vi "convertFromString.vi"(0 "reference in":refnum<class "Notification Controller.lvclass">, 5 "dateString":string, 7 "ICU?":bool, 9 "getDate":bool, 11 "error in (no error)":errorcluster, 12 "yearly?":bool, 13 "k4b2?":bool) -> (4 "reference out":refnum<class "Notification Controller.lvclass">, 6 "date":timestamp, 10 "send?":bool, 15 "error out":errorcluster)   [LabVIEW 2014, in "Notification Controller.lvclass"]
uses:
  Notification Controller.lvclass
  <vilib>/Utility/miscctls.llb/LVDateTimeRec.ctl
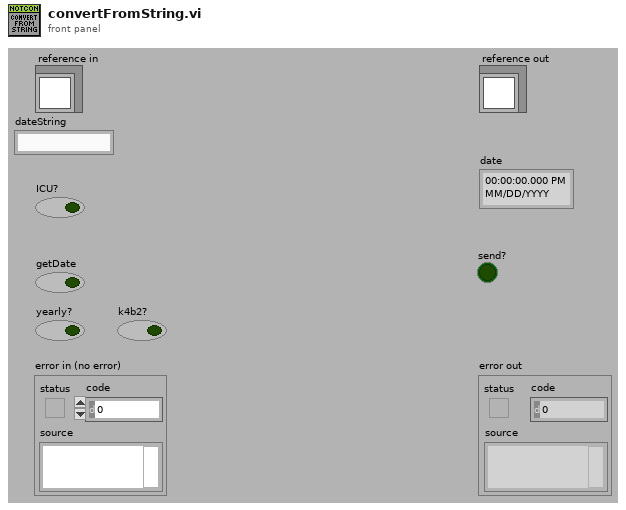
[diagram p1: front panel]
types:
  T1 = cluster{"second":i32, "minute":i32, "hour":i32, "day of month":i32, "month":i32, "year":i32, "day of week":i32, "day of year":i32, "is DST":i32}
  T2 = typedef "LVDateTimeRec.ctl" = cluster{"fractional second":dbl, "second":i32, "minute":i32, "hour":i32, "day of month":i32, "month":i32, "year":i32, "day of week":i32, "day of year":i32, "DST":i32}
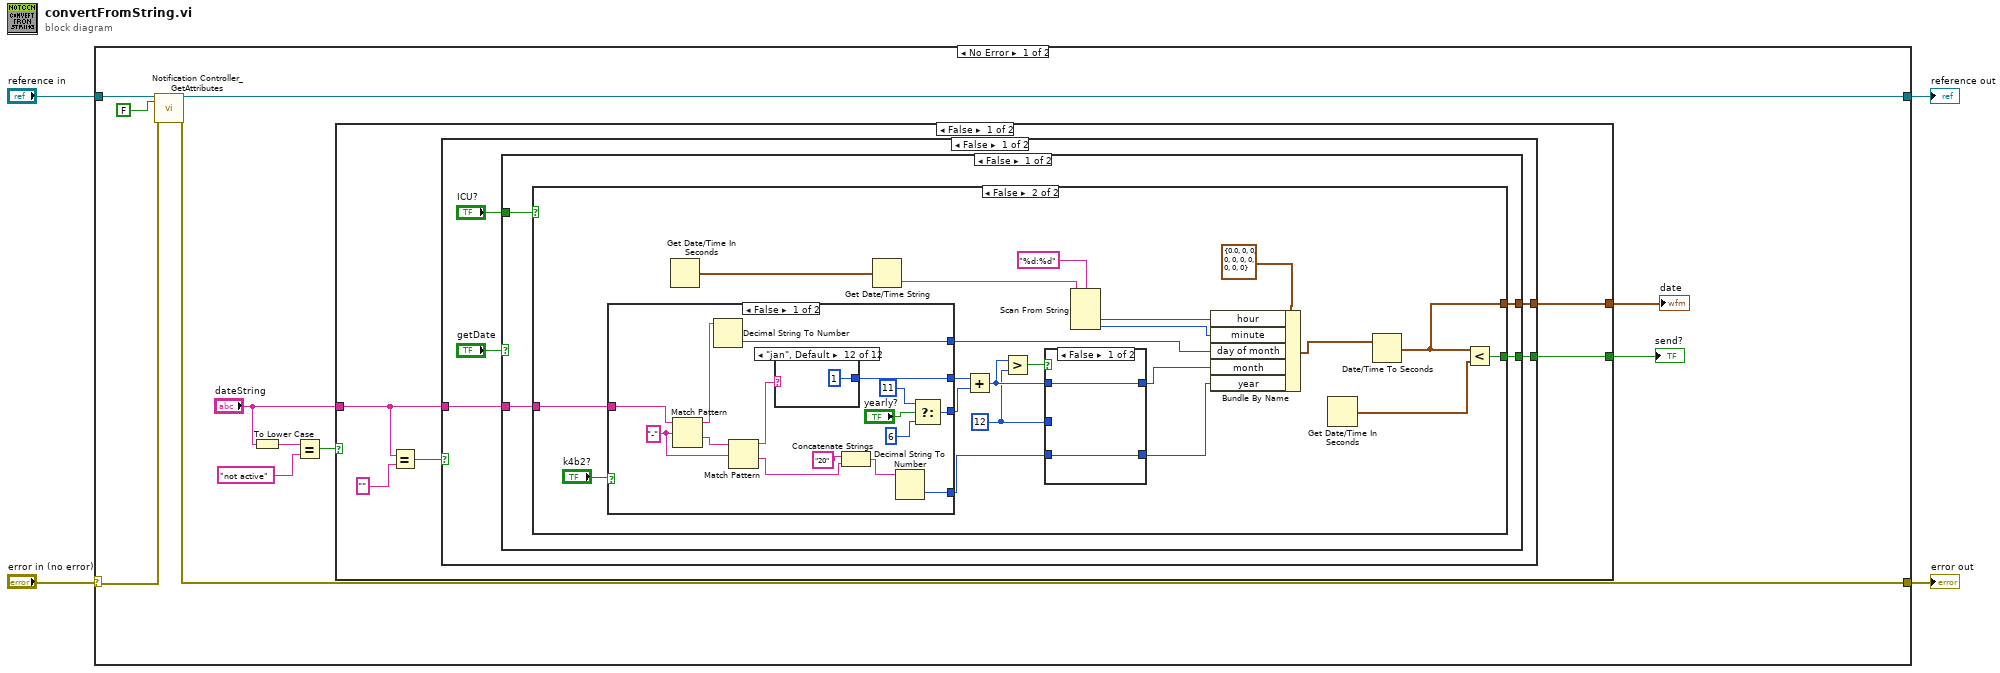
[diagram p0: block diagram]
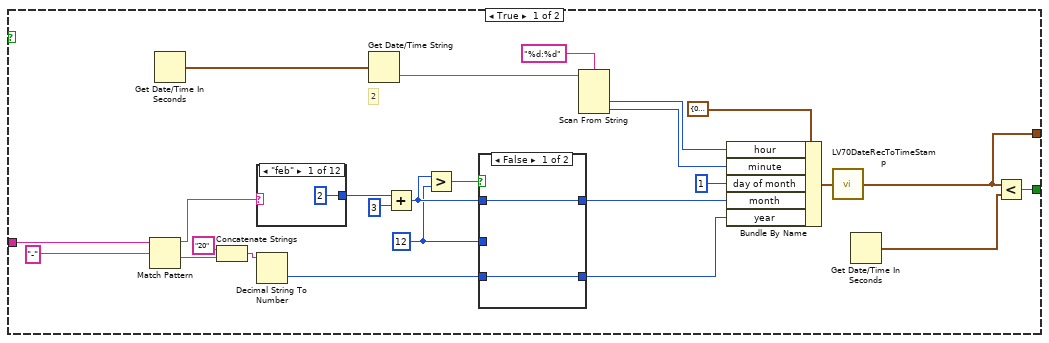
[diagram p2: hidden frame]
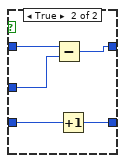
[diagram p3: hidden frame]
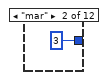
[diagram p4: hidden frame]
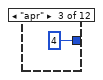
[diagram p5: hidden frame]
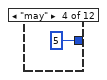
[diagram p6: hidden frame]
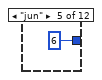
[diagram p7: hidden frame]
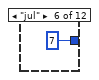
[diagram p8: hidden frame]
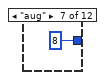
[diagram p9: hidden frame]
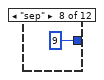
[diagram p10: hidden frame]
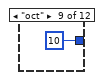
[diagram p11: hidden frame]
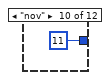
[diagram p12: hidden frame]
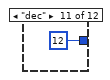
[diagram p13: hidden frame]
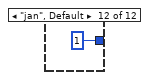
[diagram p14: hidden frame]
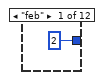
[diagram p15: hidden frame]
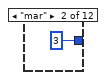
[diagram p16: hidden frame]
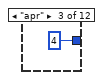
[diagram p17: hidden frame]
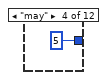
[diagram p18: hidden frame]
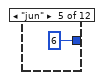
[diagram p19: hidden frame]
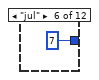
[diagram p20: hidden frame]
diagram:
  n1 = case shown="No Error" "error in (no error)" {
    selector: "error in (no error)" -> [w13 w188]
    tunnel: [w11 w188] -> w3
    tunnel: [w12 w187] -> w1
    tunnel: "reference in" -> [w15 w187]
    frame No Error {
      n2 = call "Notification Controller_GetAttributes.vi"("reference in"=w15, "return data? (T)"=FALSE, "error in (no error)"=w13) -> ("reference out"=w12:refnum<class "Notification Controller.lvclass">, "error out"=w11:errorcluster)  [unwired: 13 in, 2 out]
      n3 = To Lower Case(string="dateString") -> (all lower case string=w9:string)
      n4 = Equal?(x=w9, y="not active") -> (x = y?=w7:bool)
      n5 = case shown="False" w7 {
        tunnel: "dateString" -> [w19 _]
        tunnel: [w17 timestamp(0 s since 1904-01-01) ("Time Stamp")] -> w6
        tunnel: [w16 FALSE] -> w5
        frame False {
          n6 = Equal?(x=w19, y="") -> (x = y?=w18:bool)
          n7 = case shown="False" w18 {
            tunnel: [w24 TRUE] -> w16
            tunnel: [w23 timestamp(0 s since 1904-01-01) ("Time Stamp")] -> w17
            tunnel: w19 -> [w21 _]
            frame False {
              n8 = case shown="False" "getDate" {
                tunnel: w21 -> [w29 w157]
                tunnel: "ICU?" -> [w28 _]
                tunnel: [w27 FALSE] -> w24
                tunnel: [w26 w154] -> w23
                frame False {
                  n9 = case shown="False" w28 {
                    tunnel: w29 -> [w39 w83]
                    tunnel: [w34 w89] -> w27
                    tunnel: [w33 w77] -> w26
                    frame True {
                      w43 = 12 ("y")
                      # "2"
                      n10 = Match Pattern(string=w39, regular expression="-") -> (before substring=w37:string, after substring=w31:string)  [unwired: 1 in, 2 out]
                      n11 = Get Date/Time In Seconds() -> (seconds since 1Jan1904=w54:timestamp)
                      n12 = Concatenate Strings("20" ("string"), w31) -> (w30:string)
                      n13 = case shown="\"feb\"" w37 {
                        tunnel: [2 ("month") 3 ("month") 4 ("month") 5 ("month") 6 ("month") 7 ("month") 8 ("month") 9 ("month") 10 ("month") 11 ("month") 12 ("month") 1 ("month")] -> w47
                        frame "feb" {
                        }
                        frame "mar" {
                        }
                        frame "apr" {
                        }
                        frame "may" {
                        }
                        frame "jun" {
                        }
                        frame "jul" {
                        }
                        frame "aug" {
                        }
                        frame "sep" {
                        }
                        frame "oct" {
                        }
                        frame "nov" {
                        }
                        frame "dec" {
                        }
                        frame "jan", Default {
                        }
                      }
                      n14 = Decimal String To Number(string=w30) -> (number=w36:i32)  [unwired: 2 in, 1 out]
                      n15 = Get Date/Time String(seconds (now)=w54) -> (time string=w48:string)  [unwired: 3 out]
                      n16 = Add(x=w47, y=3) -> (x+y=w44:i32)
                      n17 = Greater?(x=w44, y=w43) -> (0:w45:bool)
                      n18 = case shown="False" w45 {
                        tunnel: w36 -> [w55 w59]
                        tunnel: w44 -> [w56 w61]
                        tunnel: w43 -> [_ w60]
                        tunnel: [w55 w57] -> w41
                        tunnel: [w56 w58] -> w42
                        frame False {
                        }
                        frame True {
                          n19 = Subtract(x=w61, y=w60) -> (x-y=w58:i32)
                          n20 = Increment(x=w59) -> (x+1=w57:i32)
                        }
                      }
                      n21 = Scan From String "Scan From String"(format string="%d:%d", input string=w48) -> (output 1=w50:i32, output 2=w49:i32)  [unwired: 4 in, 3 out]
                      n22 = Bundle By Name(cluster=T1 {"second"=0, "minute"=0, "hour"=0, "day of month"=0, "month"=0, "year"=0, "day of week"=0, "day of year"=0, "is DST"=0} ("date time rec"), "hour"=w50, "minute"=w49, "day of month"=1, "month"=w42, "year"=w41) -> (w51:T1)
                      n23 = call <vilib>:"LV70DateRecToTimeStamp.vi"("date time rec"=w51) -> ("Time Stamp"=w33:timestamp)
                      n24 = Get Date/Time In Seconds() -> (seconds since 1Jan1904=w35:timestamp)
                      n25 = Less?(x=w33, y=w35) -> (x < y?=w34:bool)
                    }
                    frame False {
                      w85 = 12 ("y")
                      n26 = case shown="False" "k4b2?" {
                        tunnel: [w109 w131] -> w88
                        tunnel: [w108 w130] -> w84
                        tunnel: w83 -> [w107 w129]
                        tunnel: [w103 11 ("y")] -> w80
                        tunnel: [w95 1] -> w75
                        frame False {
                          w99 = "-" ("regular expression")
                          n27 = Match Pattern(string=w107, regular expression=w99) -> (before substring=w96:string, after substring=w100:string)  [unwired: 1 in, 2 out]
                          n28 = Decimal String To Number(string=w96) -> (number=w95:i32)  [unwired: 2 in, 1 out]
                          n29 = Match Pattern(string=w100, regular expression=w99) -> (before substring=w98:string, after substring=w97:string)  [unwired: 1 in, 2 out]
                          n30 = case shown="\"jan\", Default" w98 {
                            tunnel: [2 ("month") 3 ("month") 4 ("month") 5 ("month") 6 ("month") 7 ("month") 8 ("month") 9 ("month") 10 ("month") 11 ("month") 12 ("month") 1 ("month")] -> w109
                            frame "feb" {
                            }
                            frame "mar" {
                            }
                            frame "apr" {
                            }
                            frame "may" {
                            }
                            frame "jun" {
                            }
                            frame "jul" {
                            }
                            frame "aug" {
                            }
                            frame "sep" {
                            }
                            frame "oct" {
                            }
                            frame "nov" {
                            }
                            frame "dec" {
                            }
                            frame "jan", Default {
                            }
                          }
                          n31 = Concatenate Strings("20" ("string"), w97) -> (w102:string)
                          n32 = Decimal String To Number(string=w102) -> (number=w108:i32)  [unwired: 2 in, 1 out]
                          n33 = Select(t=11 ("y"), s="yearly?", f=6 ("y")) -> (s? t:f=w103:i32)
                        }
                        frame True {
                          n34 = Match Pattern(string=w129, regular expression="-") -> (before substring=w124:string, after substring=w125:string)  [unwired: 1 in, 2 out]
                          n35 = case shown="\"jan\", Default" w124 {
                            tunnel: [2 ("month") 3 ("month") 4 ("month") 5 ("month") 6 ("month") 7 ("month") 8 ("month") 9 ("month") 10 ("month") 11 ("month") 12 ("month") 1 ("month")] -> w131
                            frame "feb" {
                            }
                            frame "mar" {
                            }
                            frame "apr" {
                            }
                            frame "may" {
                            }
                            frame "jun" {
                            }
                            frame "jul" {
                            }
                            frame "aug" {
                            }
                            frame "sep" {
                            }
                            frame "oct" {
                            }
                            frame "nov" {
                            }
                            frame "dec" {
                            }
                            frame "jan", Default {
                            }
                          }
                          n36 = Concatenate Strings("20" ("string"), w125) -> (w128:string)
                          n37 = Decimal String To Number(string=w128) -> (number=w130:i32)  [unwired: 2 in, 1 out]
                        }
                      }
                      n38 = Get Date/Time In Seconds() -> (seconds since 1Jan1904=w94:timestamp)
                      n39 = Get Date/Time String(seconds (now)=w94) -> (time string=w76:string)  [unwired: 3 out]
                      n40 = Add(x=w88, y=w80) -> (x+y=w86:i32)
                      n41 = Greater?(x=w86, y=w85) -> (0:w87:bool)
                      n42 = case shown="False" w87 {
                        tunnel: w84 -> [w144 w148]
                        tunnel: w86 -> [w145 w150]
                        tunnel: w85 -> [_ w149]
                        tunnel: [w144 w146] -> w81
                        tunnel: [w145 w147] -> w82
                        frame False {
                        }
                        frame True {
                          n43 = Subtract(x=w150, y=w149) -> (x-y=w147:i32)
                          n44 = Increment(x=w148) -> (x+1=w146:i32)
                        }
                      }
                      n45 = Scan From String "Scan From String"(format string="%d:%d", input string=w76) -> (output 1=w92:i32, output 2=w91:i32)  [unwired: 4 in, 3 out]
                      n46 = Bundle By Name(cluster=T2 {"fractional second"=0.0, "second"=0, "minute"=0, "hour"=0, "day of month"=0, "month"=0, "year"=0, "day of week"=0, "day of year"=0, "DST"=0} ("date time rec"), "hour"=w92, "minute"=w91, "day of month"=w75, "month"=w82, "year"=w81) -> (w78:T2)
                      n47 = Get Date/Time In Seconds() -> (seconds since 1Jan1904=w90:timestamp)
                      n48 = Date/Time To Seconds(2:w78) -> (0:w77:timestamp)  [unwired: 1 in]
                      n49 = Less?(x=w77, y=w90) -> (x < y?=w89:bool)
                    }
                  }
                }
                frame True {
                  w161 = "-" ("regular expression")
                  n50 = Get Date/Time In Seconds() -> (seconds since 1Jan1904=w170:timestamp)
                  n51 = Get Date/Time String(seconds (now)=w170) -> (time string=w164:string)  [unwired: 3 out]
                  n52 = Match Pattern(string=w157, regular expression=w161) -> (before substring=w159:string, after substring=w158:string)  [unwired: 1 in, 2 out]
                  n53 = Decimal String To Number(string=w159) -> (number=w160:i32)  [unwired: 2 in, 1 out]
                  n54 = Match Pattern(string=w158, regular expression=w161) -> (before substring=w163:string, after substring=w151:string)  [unwired: 1 in, 2 out]
                  n55 = Scan From String "Scan From String"(format string="%d:%d", input string=w164) -> (output 1=w166:i32, output 2=w165:i32)  [unwired: 4 in, 3 out]
                  n56 = case shown="\"jan\", Default" w163 {
                    tunnel: [2 ("month") 3 ("month") 4 ("month") 5 ("month") 6 ("month") 7 ("month") 8 ("month") 9 ("month") 10 ("month") 11 ("month") 12 ("month") 1 ("month")] -> w162
                    frame "feb" {
                    }
                    frame "mar" {
                    }
                    frame "apr" {
                    }
                    frame "may" {
                    }
                    frame "jun" {
                    }
                    frame "jul" {
                    }
                    frame "aug" {
                    }
                    frame "sep" {
                    }
                    frame "oct" {
                    }
                    frame "nov" {
                    }
                    frame "dec" {
                    }
                    frame "jan", Default {
                    }
                  }
                  n57 = Concatenate Strings("20" ("string"), w151) -> (w152:string)
                  n58 = Decimal String To Number(string=w152) -> (number=w156:i32)  [unwired: 2 in, 1 out]
                  n59 = Bundle By Name(cluster=T1 {"second"=0, "minute"=0, "hour"=0, "day of month"=0, "month"=0, "year"=0, "day of week"=0, "day of year"=0, "is DST"=0} ("date time rec"), "hour"=w166, "minute"=w165, "day of month"=w160, "month"=w162, "year"=w156) -> (w167:T1)
                  n60 = call <vilib>:"LV70DateRecToTimeStamp.vi"("date time rec"=w167) -> ("Time Stamp"=w154:timestamp)
                }
              }
            }
            frame True {
            }
          }
        }
        frame True {
        }
      }
      "send?" <- w5
      "date" <- w6
    }
    frame Error {
    }
  }
  "error out" <- w3
  "reference out" <- w1
